vi "Test LUnit Verify.vi"(11 "Test Case In":refnum<class "Extension Error Propagation Tests.lvclass">) -> (0 "error out":errorcluster, 3 "Test Case Out":refnum<class "Extension Error Propagation Tests.lvclass">)   [LabVIEW 2020, in "Extension Error Propagation Tests.lvclass"]
uses:
  Extension Error Propagation Tests.lvclass
  Source/Approval Tests/Options/Options.lvclass/Options.ctl
  Source/Approval Tests/Naming Data/Naming Data.lvclass/Naming Data.ctl
  <vilib>/Astemes/LUnit/Test Case.lvclass/Test Case.ctl
  Source/Approval Tests/Scrubber/Scrubber.lvclass
  Source/Approval Tests/Namer/Namer.lvclass
  Source/Approval Tests/Naming Data/Naming Data.lvclass
  Source/Approval Tests/Reporter/Reporter.lvclass
  Source/Approval Tests/Text Comparator/Text Comparator.lvclass
  <vilib>/Comparison/Equal/Equal Functor/Equal Functor.lvclass
  Extension Error Propagation Tests.lvclass/Extension Error Propagation Tests.ctl
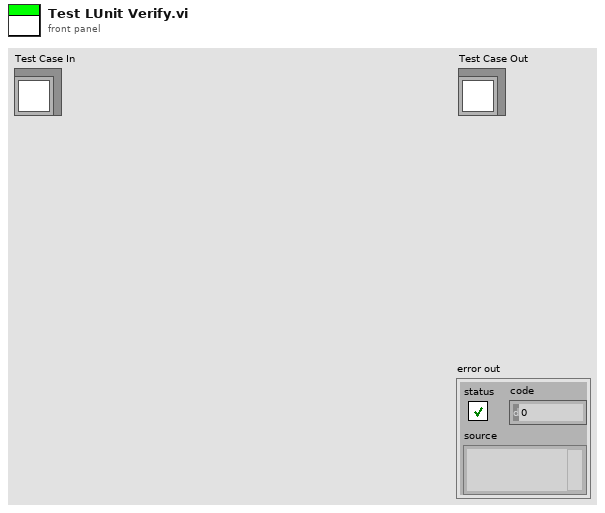
[diagram p1: front panel]
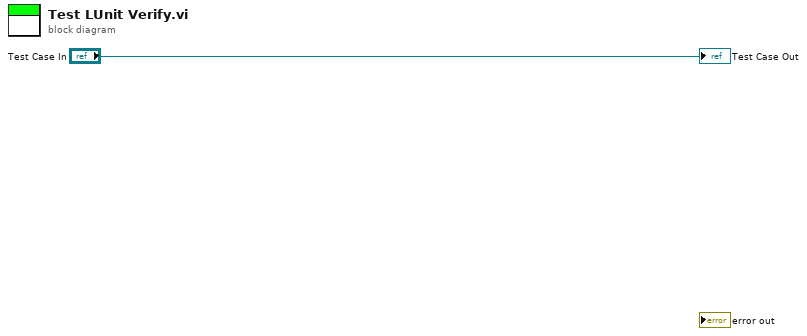
[diagram p0: block diagram]
diagram:
  "Test Case Out" <- "Test Case In"
